vi "set file meta.vi"(8 "error in (no error)":errorcluster, 11 "5785_3.2GHz_one channel in":refnum<class "5785_3.2GHz_one channel.lvclass">) -> (0 "error out":errorcluster, 3 "5785_3.2GHz_one channel out":refnum<class "5785_3.2GHz_one channel.lvclass">)   [LabVIEW 2021, in "5785_3.2GHz_one channel.lvclass"]
uses:
  5785_3.2GHz_one channel.lvclass
  pulse_tx_vis/device_mode.ctl
  5785_3.2GHz_one channel.lvclass/5785_3.2GHz_one channel.ctl
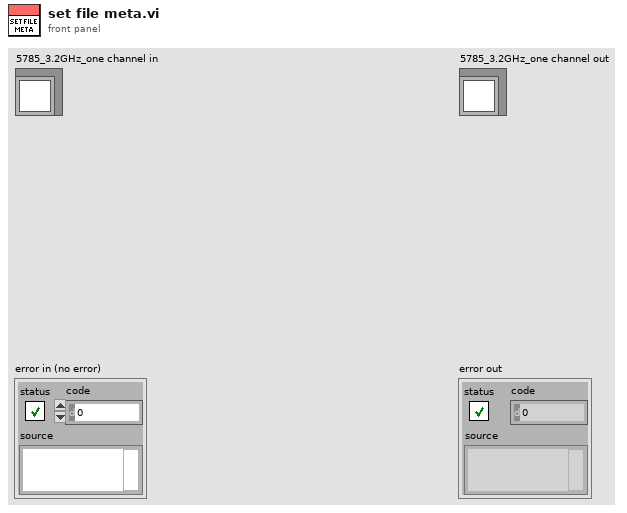
[diagram p1: front panel]
types:
  T1 = typedef "device_mode.ctl" = enum16{"USRP - 180MHz", "5785 - 2*180MHz", "5785 - 3.2GHz", "P2P - VST"}
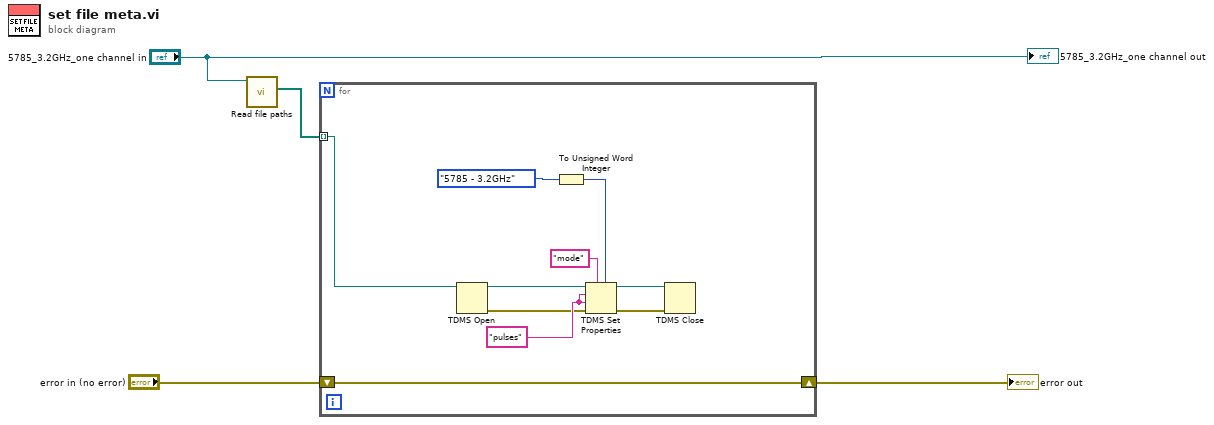
[diagram p0: block diagram]
diagram:
  n1 = call-dynamic "Read file paths.vi"("device_type in"="5785_3.2GHz_one channel in") -> ("file paths"=w4:path[])  [unwired: 8 in, 2 out]
  n2 = for {
    tunnel: w4 -> [w11] mode=indexing
    shift-right: [w14] -> w2
    shift-left: "error in (no error)" -> [w14]
    w13 = "pulses" ("channel name")
    n3 = TDMS Open(11:w11) -> (0:w8:errorcluster, 3:w12:refnum<k34>)  [unwired: 6 in]
    n4 = To Unsigned Word Integer(number=device_mode."5785 - 3.2GHz" ("Mode")) -> (unsigned 16bit integer=w5:u16)
    n5 = TDMS Set Properties(5:w5, 7:"mode", 8:w8, 9:w13, 10:w13, 11:w12) -> (0:w9:errorcluster, 3:w10:refnum<k34>)  [unwired: 2 out]
    n6 = TDMS Close(8:w9, 11:w10) -> ()  [unwired: 2 out]
  }
  "error out" <- w2
  "5785_3.2GHz_one channel out" <- "5785_3.2GHz_one channel in"
